vi "West Equation.vi"(10 "O2%":dbl=20.94, 11 "P (mb)":dbl) -> (3 "Altitude (m)":dbl)   [LabVIEW 2013]
doc: "This is a model of the atmospere based on the work of John West which defines a barometric pressure as a function of altitude. The equation is quadratic:\n\nPb = exp(6.63268-0.1112h-0.00149h^2)\n\nwhere Pb is the baromtetric pressure in mmHg and h is the altitude in meters."
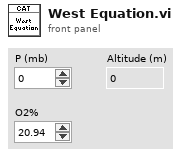
[diagram p1: front panel]
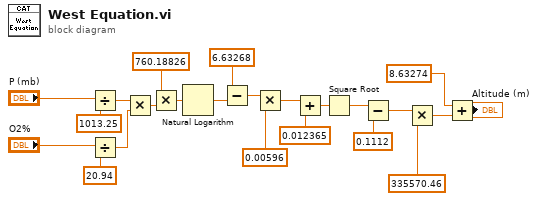
[diagram p0: block diagram]
diagram:
  n1 = Divide(x="P (mb)", y=1013.25) -> (x/y=w5:dbl)
  n2 = Divide(x="O2%", y=20.94) -> (x/y=w4:dbl)
  n3 = Multiply(x=w5, y=w4) -> (x*y=w8:dbl)
  n4 = Multiply(x=760.18826, y=w8) -> (x*y=w9:dbl)
  n5 = Natural Logarithm(1:w9) -> (0:w11:dbl)
  n6 = Subtract(x=6.63268, y=w11) -> (x-y=w12:dbl)
  n7 = Multiply(x=w12, y=0.00596 ("x")) -> (x*y=w14:dbl)
  n8 = Add(x=w14, y=0.012365 ("x")) -> (x+y=w16:dbl)
  n9 = Square Root(x=w16) -> (sqrt(x)=w17:dbl)
  n10 = Subtract(x=w17, y=0.1112 ("x")) -> (x-y=w19:dbl)
  n11 = Multiply(x=w19, y=335570.46 ("x")) -> (x*y=w21:dbl)
  n12 = Add(x=8.63274, y=w21) -> (x+y=→"Altitude (m)":dbl)
